vi "Write Voltage.AV.vi"(8 "error in":errorcluster, 10 "Voltage.AV":dbl, 11 "Cycler in":refnum<class "Cycler.lvclass">) -> (0 "error out":errorcluster, 3 "Cycler out":refnum<class "Cycler.lvclass">)   [LabVIEW 2023, in "Cycler.lvclass"]
uses:
  Cycler.lvclass
  Cycler.lvclass/Cycler.ctl
  <vilib>/ADAS Replay HIL/Channels/Tag Wrapper/Polymorphic/Write Channel (Double).vi/cccb8e89-591f-4bb4-9d4e-ae06ba1f5498.vi
  <vilib>/ADAS Replay HIL/Channels/Tag Wrapper/Polymorphic/Write Channel (Double).vi/cccb8e89-591f-4bb4-9d4e-ae06ba1f5498.vi/4bc1c15b-36ab-481f-b8dd-c64075ce723a.vi
  <vilib>/ADAS Replay HIL/Channels/Tag Wrapper/Polymorphic/Write Channel (Double).vi/cccb8e89-591f-4bb4-9d4e-ae06ba1f5498.vi/d83cb72b-7713-41fc-a3d1-682de79cf574.vi
  <vilib>/ADAS Replay HIL/Channels/Tag Wrapper/Polymorphic/Write Channel (Double).vi
  <vilib>/ADAS Replay HIL/Channels/Tag Wrapper/Tag Wrapper.lvlib
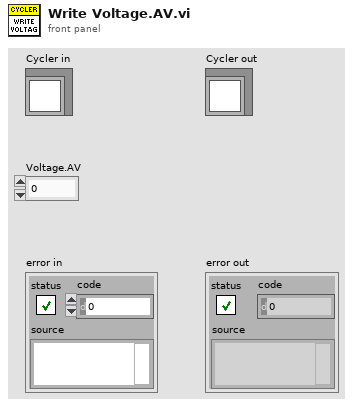
[diagram p1: front panel]
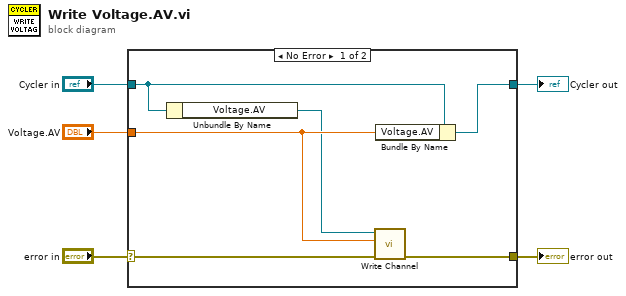
[diagram p0: block diagram]
diagram:
  n1 = case shown="No Error" "error in" {
    selector: "error in" -> [w10 w12]
    tunnel: [w9 w12] -> w4
    tunnel: [w11 w13] -> w2
    tunnel: "Cycler in" -> [w7 w13]
    tunnel: "Voltage.AV" -> [w8 _]
    frame No Error {
      n2 = Unbundle By Name(w7) -> ("Voltage.AV"=w6:refnum<k21>)
      n3 = call-poly <vilib>:"Write Channel.vi"("error in"=w10, "Value to Write"=w8, "ADAS HIL Channel in"=w6) -> ("error out"=w9:errorcluster)  [unwired: 6 in, 2 out]
      n4 = Bundle By Name(cluster=w7, "Voltage.AV"=w8) -> (w11:refnum<class "Cycler.lvclass">)
    }
    frame Error {
    }
  }
  "error out" <- w4
  "Cycler out" <- w2
